vi "Execute.vi"(8 "error in (no error)":errorcluster, 10 "Context in":refnum<class "Context.lvclass">, 11 "Stop Constant Query Command in":refnum<class "Stop Constant Query Command.lvclass">) -> (0 "error out":errorcluster, 2 "Context out":refnum<class "Context.lvclass">, 3 "Stop Constant Query Command out":refnum<class "Stop Constant Query Command.lvclass">)   [LabVIEW 2016, in "Stop Constant Query Command.lvclass"]
uses:
  Stop Constant Query Command.lvclass
  Context/Context.lvclass
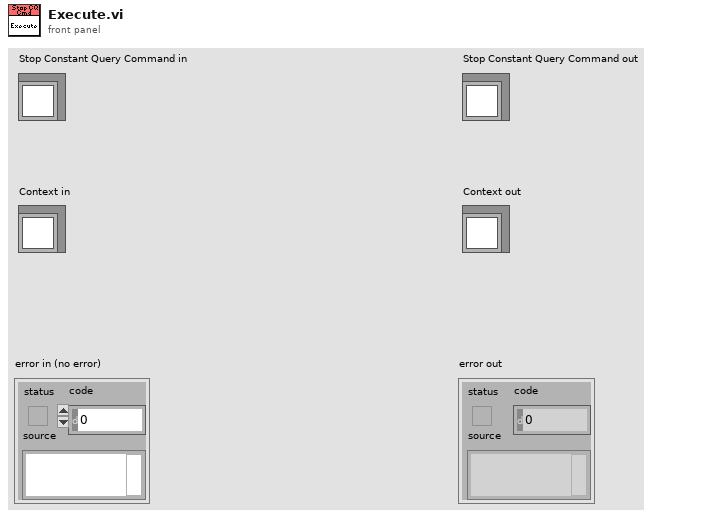
[diagram p1: front panel]
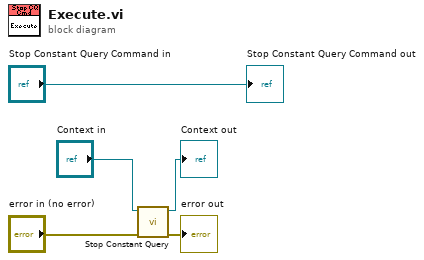
[diagram p0: block diagram]
diagram:
  n1 = call "Stop Constant Query.vi"("error in (no error)"="error in (no error)", "Context in"="Context in") -> ("error out"=→"error out":errorcluster, "Context out"=→"Context out":refnum<class "Context.lvclass">)  [unwired: 8 in]
  "Stop Constant Query Command out" <- "Stop Constant Query Command in"
